vi "State_Machine.vi"(8 "error in (no error)":errorcluster caption="entrée d'erreur (pas d'erreur)", 11 "Get_Voltage en entrée":refnum<class "Nodon_Stop_Calibration_RS.lvclass">) -> (0 "error out":errorcluster caption="sortie d'erreur", 2 "Json_String":string, 3 "Get_Voltage en sortie":refnum<class "Nodon_Stop_Calibration_RS.lvclass">)   [LabVIEW 2020, in "Library Test.lvlib" / "Nodon_Stop_Calibration_RS.lvclass"]
uses:
  Nodon_Stop_Calibration_RS.lvclass
  C:/Users/ngarcin/OneDrive - Altyor/Standard TB/Class/Test/Test (Default)/Test (Default).lvclass
  C:/Users/ngarcin/OneDrive - Altyor/Standard TB/Class/Test/Nodon_Send_Command_UART/Nodon_Send_Command_UART.lvclass
  Nodon_Send_Command_UART/Nodon_Send_Command_UART.lvclass
  Nodon_Stop_Calibration_RS.lvclass/Nodon_Stop_Calibration_RS.ctl
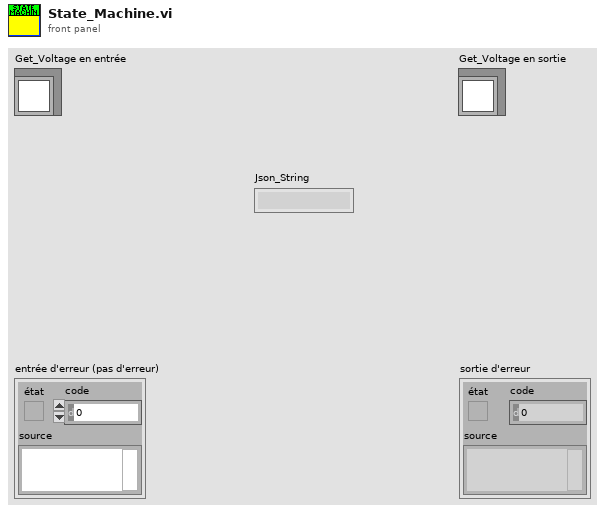
[diagram p1: front panel]
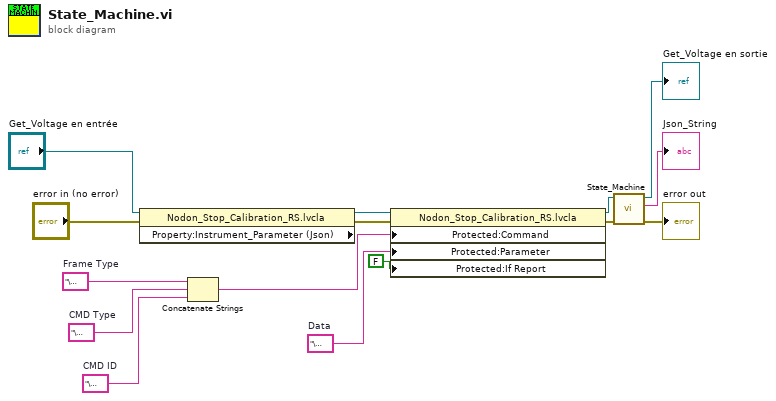
[diagram p0: block diagram]
diagram:
  w1 = "\u0002"  # Data
  w10 = "\u0000"  # Frame Type
  w9 = "\u0016"  # CMD ID
  w8 = "\u0000"  # CMD Type
  n1 = property class="Nodon_Stop_Calibration_RS.lvcla" props=["Property:Instrument_Parameter (Json)"](reference="Get_Voltage en entrée", error in="error in (no error)") -> (reference out=w4:refnum<class "Nodon_Stop_Calibration_RS.lvclass">, error out=w2:errorcluster)  [unwired: 1 out]
  n2 = Concatenate Strings(w10, w8, w9) -> (w7:string)
  n3 = property class="Nodon_Stop_Calibration_RS.lvcla"(reference=w4, error in=w2, "Protected:Command"=w7, "Protected:Parameter"=w1, "Protected:If Report"=FALSE ("If Report")) -> (reference out=w12:refnum<class "Nodon_Stop_Calibration_RS.lvclass">, error out=w11:errorcluster)
  n4 = call-parent "State_Machine.vi"("error in (no error)"=w11, "Send_Frame en entrée"=w12) -> ("error out"=→"error out":errorcluster, "Json_String"=→"Json_String":string, "Send_Frame en sortie"=→"Get_Voltage en sortie":refnum<class "Nodon_Stop_Calibration_RS.lvclass">)  [unwired: 7 in]
